vi "ClearFaults.vi"(11 "reference in":refnum<class "Stand.lvclass">) -> (3 "reference out":refnum<class "Stand.lvclass">)   [LabVIEW 2019, in "Stand.lvclass"]
uses:
  Stand.lvclass
  Stand.lvclass/Stand.ctl
  Device_class/Device.lvclass/Device.ctl
  NeedleValve_class/NeedleValve.lvclass
  C:/Users/ANENKOV_V1/Desktop/src/Device_class/Device.lvclass
  PM_Group_class/PM_Group.lvclass
  MessageInterface_class/MessageInterface.lvclass
  DA_class/DA.lvclass
  AI_class/AI.lvclass
  Device_class/Device.lvclass
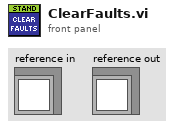
[diagram p1: front panel]
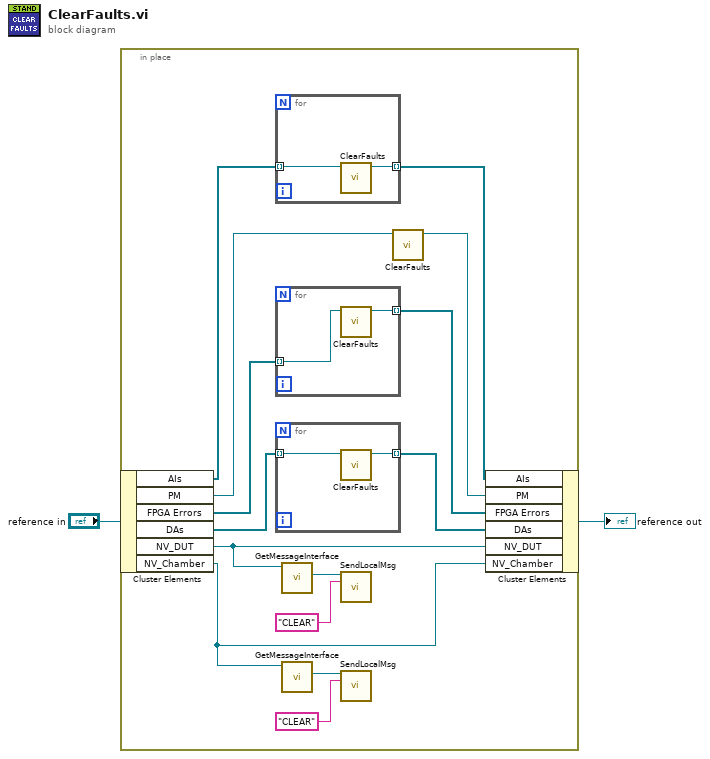
[diagram p0: block diagram]
diagram:
  n1 = in-place {
    n2 = in-place-cluster #1("reference in") -> ("AIs"=w16:refnum<class "AI.lvclass">[], "PM"=w12:refnum<class "PM_Group.lvclass">, "FPGA Errors"=w14:refnum<class "DA.lvclass">[], "DAs"=w10:refnum<class "DA.lvclass">[], "NV_DUT"=w6:refnum<class "NeedleValve.lvclass">, "NV_Chamber"=w3:refnum<class "NeedleValve.lvclass">)
    n3 = for {
      tunnel: w16 -> [w22] mode=indexing
      tunnel: [w21] -> w15 mode=indexing
      n4 = call-dynamic "ClearFaults.vi"("Sig_AI in"=w22) -> ("Sig_AI out"=w21:refnum<class "AI.lvclass">)  [unwired: 10 in]
    }
    n5 = for {
      tunnel: w14 -> [w20] mode=indexing
      tunnel: [w19] -> w13 mode=indexing
      n6 = call-dynamic "ClearFaults.vi"("DA in"=w20) -> ("DA out"=w19:refnum<class "DA.lvclass">)  [unwired: 10 in]
    }
    n7 = for {
      tunnel: w10 -> [w18] mode=indexing
      tunnel: [w17] -> w9 mode=indexing
      n8 = call-dynamic "ClearFaults.vi"("DA in"=w18) -> ("DA out"=w17:refnum<class "DA.lvclass">)  [unwired: 10 in]
    }
    n9 = call "GetMessageInterface.vi"("Device in"=w6) -> ("MessageInterface"=w8:refnum<class "MessageInterface.lvclass">)  [unwired: 10 in]
    n10 = call "GetMessageInterface.vi"("Device in"=w3) -> ("MessageInterface"=w4:refnum<class "MessageInterface.lvclass">)  [unwired: 10 in]
    n11 = call-dynamic "SendLocalMsg.vi"("reference in"=w8, "name"="CLEAR") -> ()  [unwired: 11 in, 3 out]
    n12 = call-dynamic "SendLocalMsg.vi"("reference in"=w4, "name"="CLEAR") -> ()  [unwired: 11 in, 3 out]
    n13 = call-dynamic "ClearFaults.vi"("PM_Group in"=w12) -> ("PM_Group out"=w11:refnum<class "PM_Group.lvclass">)  [unwired: 10 in]
    n14 = in-place-cluster #1("AIs"=w15, "PM"=w11, "FPGA Errors"=w13, "DAs"=w9, "NV_DUT"=w6, "NV_Chamber"=w3) -> (→"reference out":refnum<class "Stand.lvclass">)
  }
